vi "Initialize Device Core.vi"(8 "error in (no error)":errorcluster, 9 "Reset (F)":bool, 10 "Resource Name":string, 11 "CS++SimMotor in":refnum<class "CS++SimMotor.lvclass">) -> (0 "error out":errorcluster, 3 "CS++SimMotor out":refnum<class "CS++SimMotor.lvclass">)   [LabVIEW 2015, in "CS++SimMotor.lvlib" / "CS++SimMotor.lvclass"]
doc: "Initialize device driver."
uses:
  CS++SimMotor.lvclass
  CSPP_Core/Classes/CS++ProcessVariables/ProcessVariable/PV.lvclass
  CS++SimMotor.lvclass/CS++SimMotor.ctl
  CSPP_Core/Classes/CS++ProcessVariables/ProcessVariable/PV.lvclass/PV.ctl
  CSPP_Core/Classes/CS++ProcessVariables/ProcessVariable/Write Data.vi
  CSPP_Core/Classes/CS++ProcessVariables/ProcessVariable/Write Timestamp.vi
  CSPP_Core/Classes/CS++ProcessVariables/ProcessVariable/Write Quality.vi
  CSPP_Core/Classes/CS++ProcessVariables/ProcessVariable/Write status.vi
  CSPP_DeviceBase/CS++Motor/CS++Motor.lvclass
  CSPP_Core/Classes/CS++ProcessVariables/PVConnection/PVConnection.lvclass
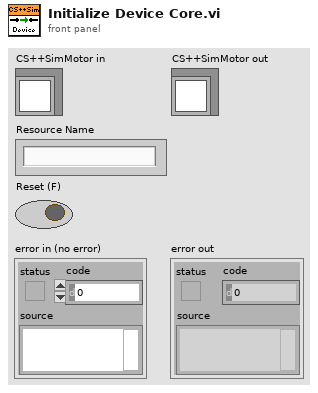
[diagram p1: front panel]
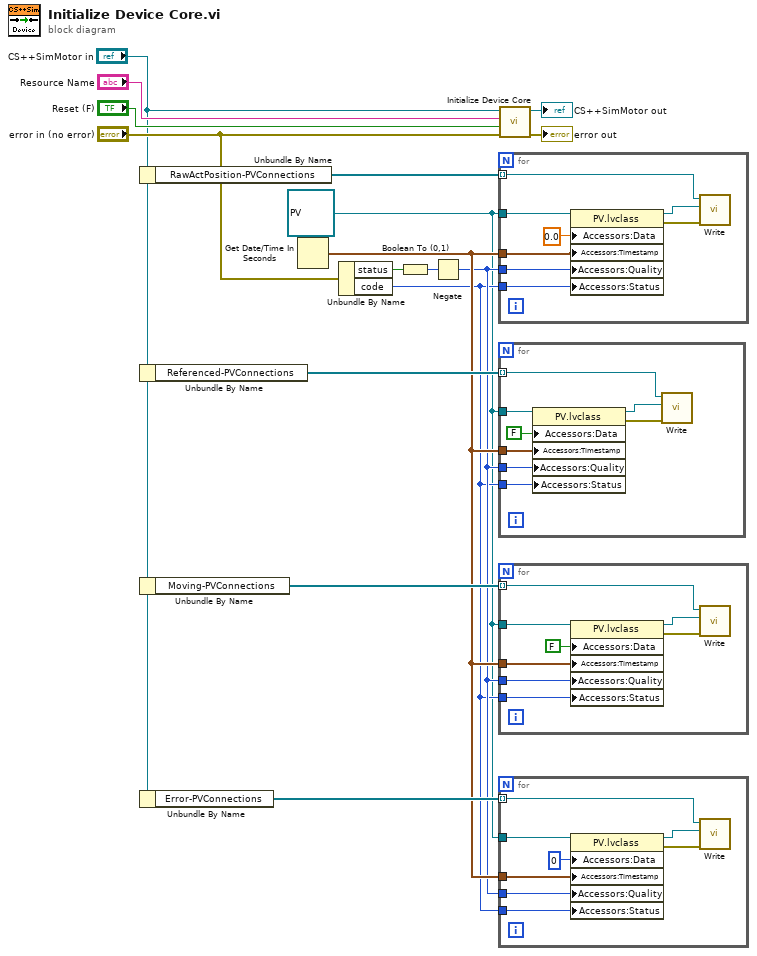
[diagram p0: block diagram]
diagram:
  w1 = refnum<class "PV.lvclass"> refnum ("PV")
  n1 = Unbundle By Name("CS++SimMotor in") -> ("RawActPosition-PVConnections"=w9:refnum<class "PVConnection.lvclass">[])
  n2 = Unbundle By Name("CS++SimMotor in") -> ("Referenced-PVConnections"=w8:refnum<class "PVConnection.lvclass">[])
  n3 = Unbundle By Name("CS++SimMotor in") -> ("Moving-PVConnections"=w7:refnum<class "PVConnection.lvclass">[])
  n4 = Unbundle By Name("CS++SimMotor in") -> ("Error-PVConnections"=w6:refnum<class "PVConnection.lvclass">[])
  n5 = Get Date/Time In Seconds() -> (seconds since 1Jan1904=w4:timestamp)
  n6 = Unbundle By Name("error in (no error)") -> ("status"=w10:bool, "code"=w2:i32)
  n7 = Boolean To (0,1)(Boolean=w10) -> (0, 1=w12:i16)
  n8 = Negate(x=w12) -> (-x=w3:i16)
  n9 = for {
    tunnel: w1 -> [w22]
    tunnel: w4 -> [w21]
    tunnel: w3 -> [w20]
    tunnel: w2 -> [w19]
    tunnel: w9 -> [w18] mode=indexing
    n10 = property class="PV.lvclass"(reference=w22, "Accessors:Data"=0.0, "Accessors:Timestamp"=w21, "Accessors:Quality"=w20, "Accessors:Status"=w19) -> (reference out=w24:refnum<class "PV.lvclass">, error out=w23:errorcluster)  [unwired: 1 in]
    n11 = call "Write.vi"("error in (no error)"=w23, "PV"=w24, "PVConnection in"=w18) -> ()  [unwired: 7 in, 2 out]
  }
  n12 = for {
    tunnel: w1 -> [w30]
    tunnel: w4 -> [w29]
    tunnel: w3 -> [w28]
    tunnel: w2 -> [w27]
    tunnel: w8 -> [w26] mode=indexing
    n13 = property class="PV.lvclass"(reference=w30, "Accessors:Data"=FALSE, "Accessors:Timestamp"=w29, "Accessors:Quality"=w28, "Accessors:Status"=w27) -> (reference out=w32:refnum<class "PV.lvclass">, error out=w31:errorcluster)  [unwired: 1 in]
    n14 = call "Write.vi"("error in (no error)"=w31, "PV"=w32, "PVConnection in"=w26) -> ()  [unwired: 7 in, 2 out]
  }
  n15 = for {
    tunnel: w1 -> [w38]
    tunnel: w4 -> [w37]
    tunnel: w3 -> [w36]
    tunnel: w2 -> [w35]
    tunnel: w7 -> [w34] mode=indexing
    n16 = property class="PV.lvclass"(reference=w38, "Accessors:Data"=FALSE, "Accessors:Timestamp"=w37, "Accessors:Quality"=w36, "Accessors:Status"=w35) -> (reference out=w40:refnum<class "PV.lvclass">, error out=w39:errorcluster)  [unwired: 1 in]
    n17 = call "Write.vi"("error in (no error)"=w39, "PV"=w40, "PVConnection in"=w34) -> ()  [unwired: 7 in, 2 out]
  }
  n18 = for {
    tunnel: w1 -> [w46]
    tunnel: w4 -> [w45]
    tunnel: w3 -> [w44]
    tunnel: w2 -> [w43]
    tunnel: w6 -> [w42] mode=indexing
    n19 = property class="PV.lvclass"(reference=w46, "Accessors:Data"=u8 0, "Accessors:Timestamp"=w45, "Accessors:Quality"=w44, "Accessors:Status"=w43) -> (reference out=w48:refnum<class "PV.lvclass">, error out=w47:errorcluster)  [unwired: 1 in]
    n20 = call "Write.vi"("error in (no error)"=w47, "PV"=w48, "PVConnection in"=w42) -> ()  [unwired: 7 in, 2 out]
  }
  n21 = call-parent "Initialize Device Core.vi"("error in (no error)"="error in (no error)", "Reset (F)"="Reset (F)", "Resource Name"="Resource Name", "CS++Motor in"="CS++SimMotor in") -> ("error out"=→"error out":errorcluster, "CS++Motor out"=→"CS++SimMotor out":refnum<class "CS++SimMotor.lvclass">)  [unwired: 6 in]
